vi "useA.vi"() -> (3 "Numeric":i32)   [LabVIEW 2011]
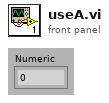
[diagram p1: front panel]
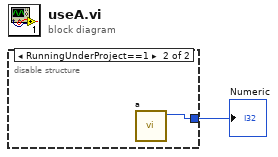
[diagram p0: block diagram]
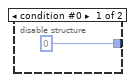
[diagram p2: hidden frame]
diagram:
  n1 = disable-structure shown="RunningUnderProject==1" {
    disable-tunnel: [0 w3] -> w1
    frame condition #0 {
    }
    frame condition #1 (active) {
      n2 = call "a.vi"() -> ("Numeric"=w3:i32)  [unwired: 11 in]
    }
  }
  "Numeric" <- w1
